vi "SetpointSequenceStateMachine.vi"(0 "VISA resource name in":refnum<visa-resource-name>, 1 "State in":i32, 5 "Section in":i32, 7 "Sweep rate":dbl, 9 "Array of X,Y,Z setpoints":dbl[][](array[numeric]), 11 "error in":errorcluster, 12 "Response in":string) -> (3 "State":i32, 4 "VISA resource name out":refnum<visa-resource-name>, 6 "Section":i32, 10 "finished":bool, 14 "Response":string, 15 "error out":errorcluster)   [LabVIEW 2013]
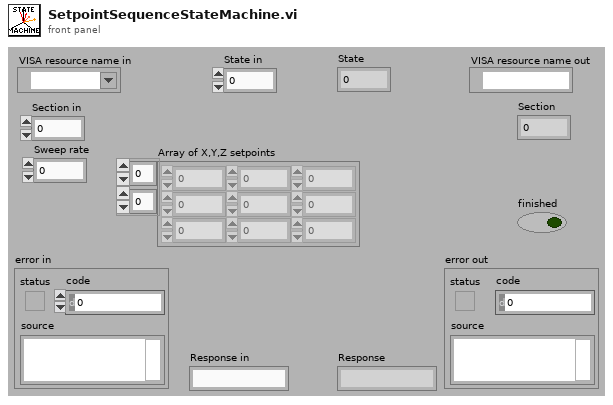
[diagram p1: front panel]
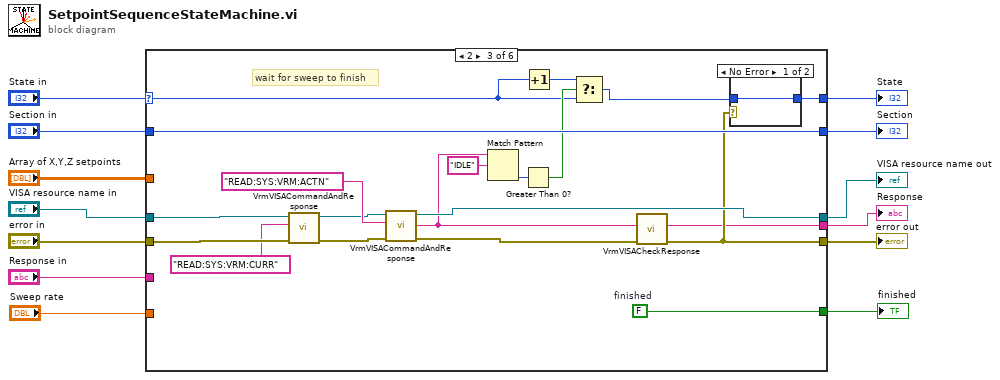
[diagram p0: block diagram]
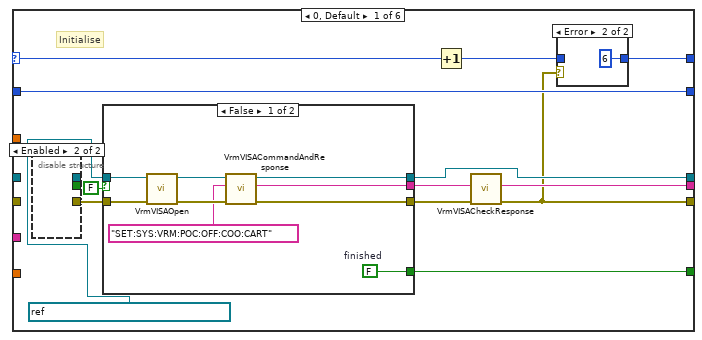
[diagram p2: hidden frame]
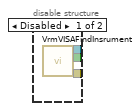
[diagram p3: hidden frame]
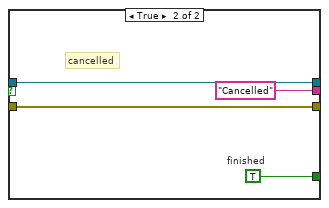
[diagram p5: hidden frame]
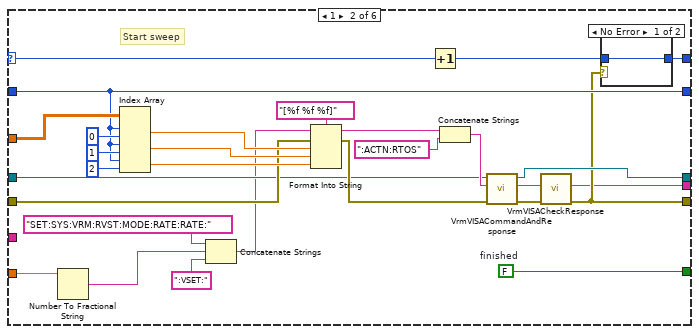
[diagram p6: hidden frame]
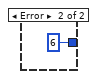
[diagram p7: hidden frame]
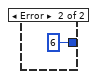
[diagram p8: hidden frame]
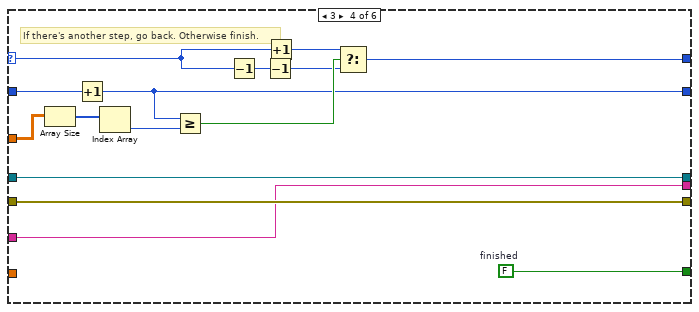
[diagram p9: hidden frame]
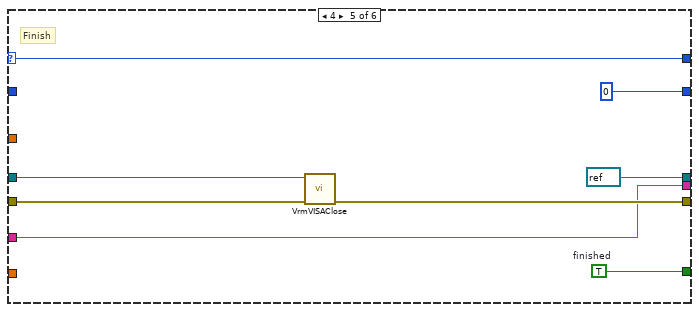
[diagram p10: hidden frame]
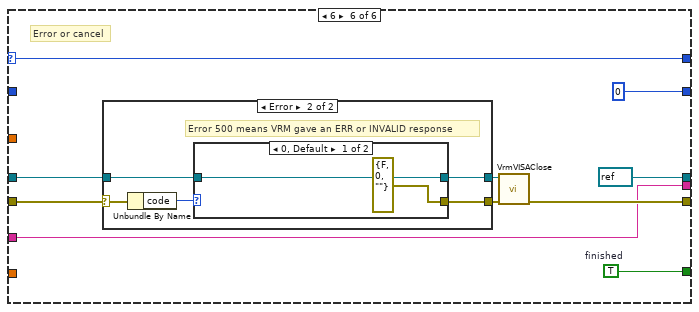
[diagram p11: hidden frame]
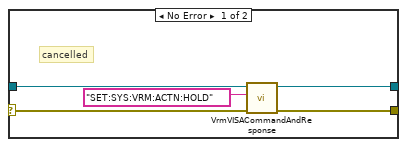
[diagram p12: hidden frame]
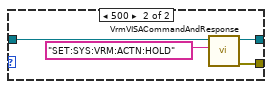
[diagram p13: hidden frame]
diagram:
  n1 = case shown="2" "State in" {
    selector: "State in" -> [w16 w54 w89 w106 w119 w129]
    tunnel: [w19 w50 w82 w101 w113 w123] -> w11
    tunnel: [w18 w52 w83 w102 w118 w128] -> w10
    tunnel: [w25 w56 w86 w107 w119 w129] -> w13
    tunnel: [w24 w65 w91 w103 refnum<visa-resource-name> refnum ("VISA resource name out") refnum<visa-resource-name> refnum ("VISA resource name out")] -> w3
    tunnel: "VISA resource name in" -> [_ w63 w80 w103 w114 w125]
    tunnel: "error in" -> [_ w64 w78 w102 w115 w121]
    tunnel: "Array of X,Y,Z setpoints" -> [_ w62 _ w112 _ _]
    tunnel: "Section in" -> [w23 w57 w95 w109 _ _]
    tunnel: [w23 w57 w95 w98 0 ("Section") 0 ("Section")] -> w9
    tunnel: [w22 w58 w87 w99 w120 w130] -> w12
    tunnel: "Response in" -> [_ _ _ w101 w113 w123]
    tunnel: "Sweep rate" -> [_ w49 _ _ _ _]
    frame 0, Default {
      # "Initialise"
      n2 = disable-structure shown="Enabled" {
        disable-tunnel: [w29 _] -> w26
        disable-tunnel: [w28 _] -> _
        disable-tunnel: [w27 _] -> _
        frame Disabled {
          n3 = call "VrmVISAFindInsrument.vi"() -> ("error out"=w29:errorcluster, "Cancelled"=w27:bool, "VISA resource name out"=w28:refnum<visa-resource-name>)  [unwired: 9 in]
        }
        frame Enabled {
        }
      }
      n4 = case shown="False" FALSE {
        tunnel: w26 -> [w37 w44]
        tunnel: refnum<visa-resource-name> "TCPIP0::127.0.0.1::33575::SOCKET" ("VISA resource name out") -> [w36 w42]
        tunnel: [w35 "Cancelled" ("Response")] -> w20
        tunnel: [w33 w44] -> w21
        tunnel: [w34 w42] -> w24
        tunnel: [w32 w41] -> w22
        frame False {
          w32 = FALSE  # finished
          n5 = call "VrmVISAOpen.vi"("error in (no error)"=w37, "VISA resource name in"=w36) -> ("error out"=w40:errorcluster, "VISA resource name out"=w39:refnum<visa-resource-name>)  [unwired: 8 in]
          n6 = call "VrmVISACommandAndResponse.vi"("error in (no error)"=w40, "Command"="SET:SYS:VRM:POC:OFF:COO:CART", "VISA resource name in"=w39) -> ("error out"=w33:errorcluster, "Response"=w35:string, "VISA resource name out"=w34:refnum<visa-resource-name>)  [unwired: 6 in]
        }
        frame True {
          w41 = TRUE  # finished
          # "cancelled"
        }
      }
      n7 = Increment(x=w16) -> (x+1=w17:i32)
      n8 = call "VrmVISACheckResponse.vi"("error in (no error)"=w21, "Response"=w20) -> ("error out"=w18:errorcluster, "Response out"=w19:string)  [unwired: 8 in]
      n9 = case shown="Error" w18 {
        tunnel: w17 -> [w30 _]
        tunnel: [w30 6] -> w25
        frame No Error {
        }
        frame Error {
        }
      }
    }
    frame 1 {
      w58 = FALSE  # finished
      # "Start sweep"
      n10 = Number To Fractional String(number=w49) -> (F-format string=w46:string)  [unwired: 3 in]
      n11 = Index Array(array=w62, index (row) #1=w57, index (col) #1=0 ("disabled index (col)"), index (row) #2=w57, index (col) #2=1 ("index (col)"), index (row) #3=w57, index (col) #3=2 ("index (col)")) -> (element #1=w67:dbl, element #2=w68:dbl, element #3=w69:dbl)
      n12 = Concatenate Strings("SET:SYS:VRM:RVST:MODE:RATE:RATE:", w46, ":VSET:") -> (w45:string)
      n13 = Format Into String(format string="[%f %f %f]", initial string=w45, error in=w64, w67, w68, w69) -> (resulting string=w71:string, error out=w72:errorcluster)
      n14 = Increment(x=w54) -> (x+1=w55:i32)
      n15 = Concatenate Strings(w71, ":ACTN:RTOS") -> (w73:string)
      n16 = call "VrmVISACommandAndResponse.vi"("error in (no error)"=w72, "Command"=w73, "VISA resource name in"=w63) -> ("error out"=w53:errorcluster, "Response"=w51:string, "VISA resource name out"=w65:refnum<visa-resource-name>)  [unwired: 6 in]
      n17 = call "VrmVISACheckResponse.vi"("error in (no error)"=w53, "Response"=w51) -> ("error out"=w52:errorcluster, "Response out"=w50:string)  [unwired: 8 in]
      n18 = case shown="No Error" w52 {
        tunnel: w55 -> [w74 _]
        tunnel: [w74 6] -> w56
        frame No Error {
        }
        frame Error {
        }
      }
    }
    frame 2 {
      w87 = FALSE  # finished
      # "wait for sweep to finish"
      n19 = call "VrmVISACommandAndResponse.vi"("error in (no error)"=w78, "Command"="READ:SYS:VRM:CURR", "VISA resource name in"=w80) -> ("error out"=w77:errorcluster, "VISA resource name out"=w79:refnum<visa-resource-name>)  [unwired: 6 in, 1 out]
      n20 = call "VrmVISACommandAndResponse.vi"("error in (no error)"=w77, "Command"="READ:SYS:VRM:ACTN", "VISA resource name in"=w79) -> ("error out"=w84:errorcluster, "Response"=w81:string, "VISA resource name out"=w91:refnum<visa-resource-name>)  [unwired: 6 in]
      n21 = Match Pattern(string=w81, regular expression="IDLE") -> (offset past match=w92:i32)  [unwired: 1 in, 3 out]
      n22 = Greater Than 0?(x=w92) -> (x > 0?=w90:bool)
      n23 = Increment(x=w89) -> (x+1=w88:i32)
      n24 = Select(t=w88, s=w90, f=w89) -> (s? t:f=w85:i32)
      n25 = call "VrmVISACheckResponse.vi"("error in (no error)"=w84, "Response"=w81) -> ("error out"=w83:errorcluster, "Response out"=w82:string)  [unwired: 8 in]
      n26 = case shown="No Error" w83 {
        tunnel: w85 -> [w96 _]
        tunnel: [w96 6] -> w86
        frame No Error {
        }
        frame Error {
        }
      }
    }
    frame 3 {
      w99 = FALSE  # finished
      # "If there's another step, go back. Otherwise finish."
      n27 = Array Size(array=w112) -> (size(s)=w111:i32[])
      n28 = Increment(x=w109) -> (x+1=w98:i32)
      n29 = Index Array(array=w111) -> (element=w110:i32)  [unwired: 1 in]
      n30 = Greater Or Equal?(x=w98, y=w110) -> (x >= y?=w108:bool)
      n31 = Decrement(x=w106) -> (x-1=w105:i32)
      n32 = Decrement(x=w105) -> (x-1=w104:i32)
      n33 = Increment(x=w106) -> (x+1=w100:i32)
      n34 = Select(t=w100, s=w108, f=w104) -> (s? t:f=w107:i32)
    }
    frame 4 {
      w120 = TRUE  # finished
      # "Finish"
      n35 = call "VrmVISAClose.vi"("error in (no error)"=w115, "VISA resource name in"=w114) -> ("error out"=w118:errorcluster)  [unwired: 9 in]
    }
    frame 6 {
      w130 = TRUE  # finished
      # "Error or cancel"
      n36 = case shown="Error" w121 {
        selector: w121 -> [w133 w140]
        tunnel: w125 -> [w134 w138]
        tunnel: [w131 w137] -> w124
        tunnel: [w132 w136] -> w122
        frame No Error {
          # "cancelled"
          n37 = call "VrmVISACommandAndResponse.vi"("error in (no error)"=w133, "Command"="SET:SYS:VRM:ACTN:HOLD", "VISA resource name in"=w134) -> ("error out"=w132:errorcluster, "VISA resource name out"=w131:refnum<visa-resource-name>)  [unwired: 6 in, 1 out]
        }
        frame Error {
          # "Error 500 means VRM gave an ERR or INVALID response"
          n38 = Unbundle By Name(w140) -> ("code"=w139:i32)
          n39 = case shown="0, Default" w139 {
            tunnel: w138 -> [w142 w145]
            tunnel: [w142 w144] -> w137
            tunnel: [errorcluster {"status"=FALSE, "code"=0, "source"=""} ("error out") w143] -> w136
            frame 0, Default {
            }
            frame 500 {
              n40 = call "VrmVISACommandAndResponse.vi"("Command"="SET:SYS:VRM:ACTN:HOLD", "VISA resource name in"=w145) -> ("error out"=w143:errorcluster, "VISA resource name out"=w144:refnum<visa-resource-name>)  [unwired: 7 in, 1 out]
            }
          }
        }
      }
      n41 = call "VrmVISAClose.vi"("error in (no error)"=w122, "VISA resource name in"=w124) -> ("error out"=w128:errorcluster)  [unwired: 9 in]
    }
  }
  "State" <- w13
  "finished" <- w12
  "Response" <- w11
  "error out" <- w10
  "Section" <- w9
  "VISA resource name out" <- w3
